vi "Wavelength2Color.vi"(8 "error in (no error)":errorcluster, 11 "Wavelength":u16=380 min=350 max=850 step=1) -> (0 "error out":errorcluster, 3 "Color":u32(colorbox))   [LabVIEW 2023]
doc: "This vi converts a wavelength into a color"
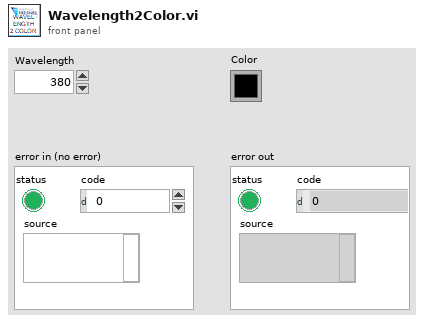
[diagram p1: front panel]
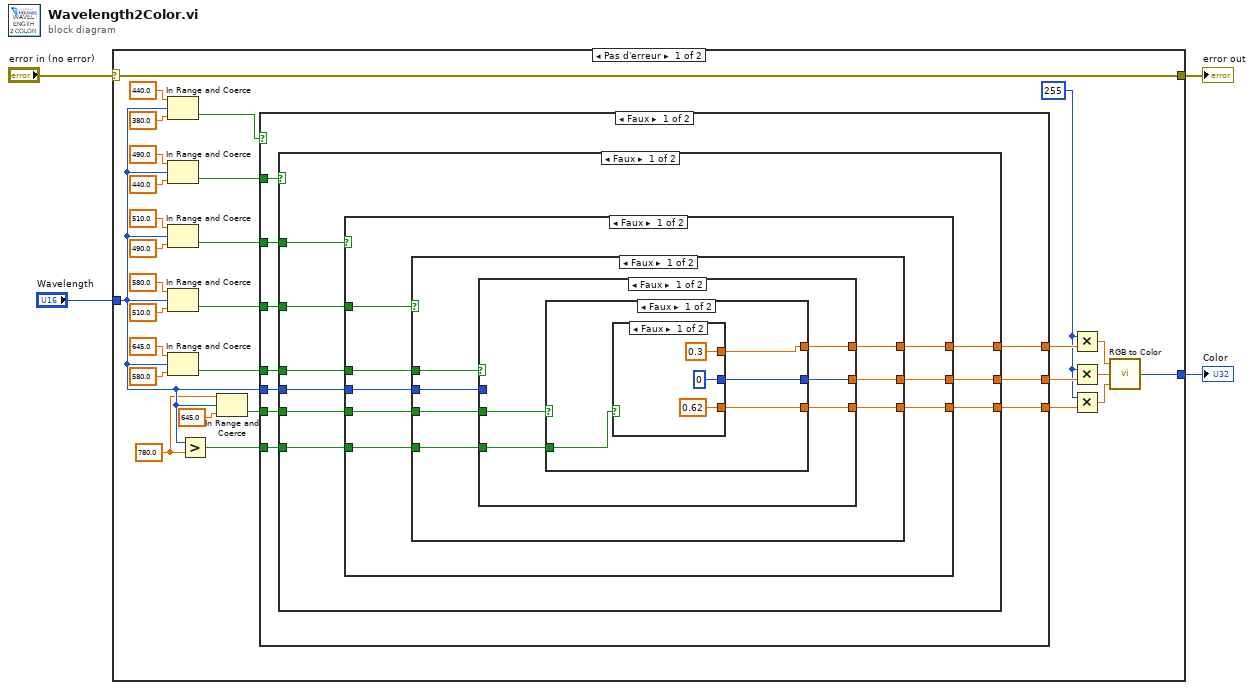
[diagram p0: block diagram]
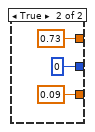
[diagram p2: hidden frame]
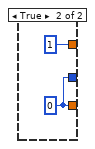
[diagram p3: hidden frame]
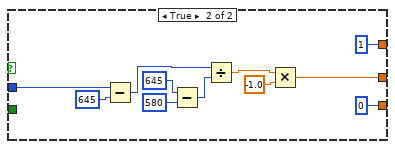
[diagram p4: hidden frame]
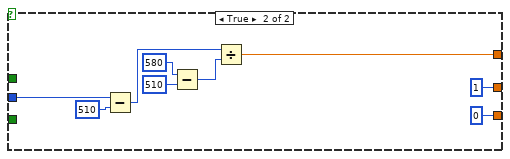
[diagram p5: hidden frame]
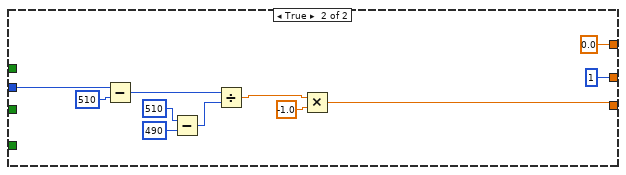
[diagram p6: hidden frame]
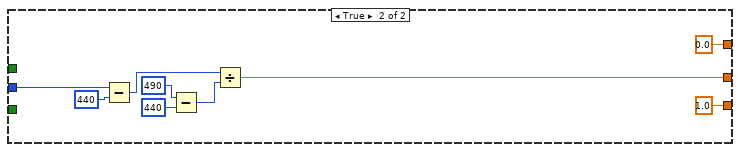
[diagram p7: hidden frame]
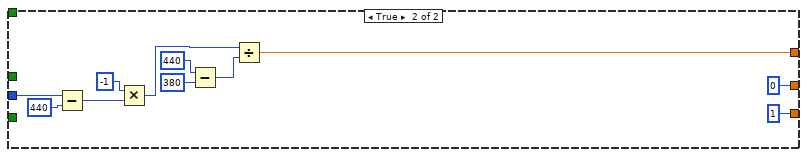
[diagram p8: hidden frame]
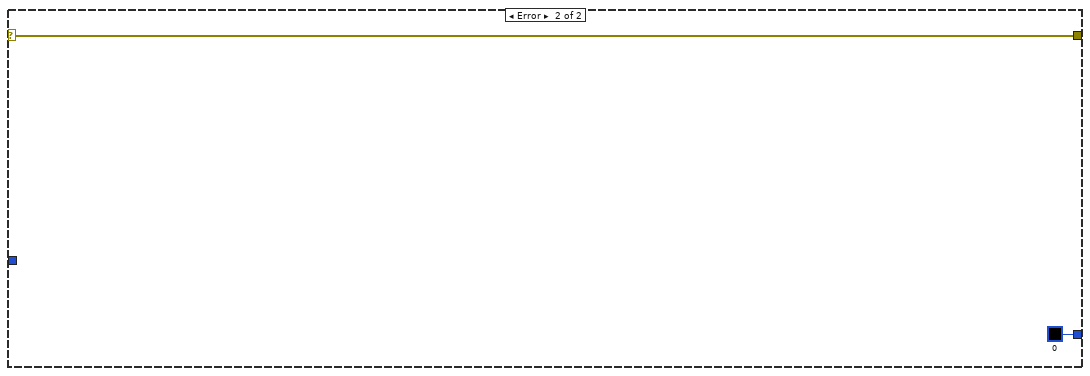
[diagram p9: hidden frame]
diagram:
  n1 = case shown="Pas d'erreur" "error in (no error)" {
    selector: "error in (no error)" -> [w8 w137]
    tunnel: [w8 w137] -> w4
    tunnel: "Wavelength" -> [w7 _]
    tunnel: [w9 u32 0 ("Color")] -> w1
    frame No Error {
      w21 = 255
      w6 = 780.0 ("upper limit")
      n2 = In Range and Coerce(upper limit=440.0, x=w7, lower limit=380.0) -> (In Range?=w22:bool)  [unwired: 1 out]
      n3 = In Range and Coerce(upper limit=490.0, x=w7, lower limit=440.0 ("upper limit")) -> (In Range?=w23:bool)  [unwired: 1 out]
      n4 = In Range and Coerce(upper limit=510.0, x=w7, lower limit=490.0 ("upper limit")) -> (In Range?=w24:bool)  [unwired: 1 out]
      n5 = In Range and Coerce(upper limit=580.0, x=w7, lower limit=510.0 ("upper limit")) -> (In Range?=w25:bool)  [unwired: 1 out]
      n6 = In Range and Coerce(upper limit=645.0, x=w7, lower limit=580.0 ("upper limit")) -> (In Range?=w26:bool)  [unwired: 1 out]
      n7 = Greater?(x=w7, y=w6) -> (0:w5:bool)
      n8 = In Range and Coerce(upper limit=w6, x=w7, lower limit=645.0 ("upper limit")) -> (In Range?=w27:bool)  [unwired: 1 out]
      n9 = case shown="Faux" w22 {
        tunnel: w23 -> [w43 _]
        tunnel: w24 -> [w42 _]
        tunnel: w25 -> [w41 _]
        tunnel: w26 -> [w40 _]
        tunnel: w27 -> [w39 _]
        tunnel: w7 -> [w35 w134]
        tunnel: [w38 w128] -> w28
        tunnel: [w36 0] -> w29
        tunnel: [w37 1] -> w30
        tunnel: w5 -> [w34 _]
        frame False {
          n10 = case shown="Faux" w43 {
            tunnel: w42 -> [w52 _]
            tunnel: w41 -> [w51 _]
            tunnel: w40 -> [w50 _]
            tunnel: w39 -> [w49 _]
            tunnel: [w48 0.0] -> w38
            tunnel: [w46 1.0] -> w37
            tunnel: [w47 w119] -> w36
            tunnel: w35 -> [w45 w118]
            tunnel: w34 -> [w44 _]
            frame False {
              n11 = case shown="Faux" w52 {
                tunnel: w51 -> [w60 _]
                tunnel: w50 -> [w59 _]
                tunnel: w49 -> [w58 _]
                tunnel: [w56 0.0] -> w48
                tunnel: [w55 1] -> w47
                tunnel: [w54 w107] -> w46
                tunnel: w45 -> [w57 w109]
                tunnel: w44 -> [w53 _]
                frame False {
                  n12 = case shown="Faux" w60 {
                    tunnel: w59 -> [w67 _]
                    tunnel: w58 -> [w66 _]
                    tunnel: w57 -> [w65 w99]
                    tunnel: [w63 w98] -> w56
                    tunnel: [w64 1] -> w55
                    tunnel: [w62 0] -> w54
                    tunnel: w53 -> [w61 _]
                    frame False {
                      n13 = case shown="Faux" w67 {
                        tunnel: w66 -> [w72 _]
                        tunnel: w65 -> [_ w89]
                        tunnel: [w70 w87] -> w64
                        tunnel: [w71 1] -> w63
                        tunnel: [w69 0] -> w62
                        tunnel: w61 -> [w68 _]
                        frame False {
                          n14 = case shown="Faux" w72 {
                            tunnel: [w73 1] -> w71
                            tunnel: [w74 w83] -> w70
                            tunnel: [w75 w83] -> w69
                            tunnel: w68 -> [w76 _]
                            frame False {
                              n15 = case shown="Faux" w76 {
                                tunnel: [0.62 0.09] -> w75
                                tunnel: [u8 0 0] -> w74
                                tunnel: [0.3 0.73] -> w73
                                frame False {
                                }
                                frame True {
                                }
                              }
                            }
                            frame True {
                              w83 = 0
                            }
                          }
                        }
                        frame True {
                          n16 = Subtract(x=w89, y=645) -> (x-y=w95:i32)
                          n17 = Subtract(x=645, y=580) -> (x-y=w93:i32)
                          n18 = Divide(x=w95, y=w93) -> (x/y=w88:dbl)
                          n19 = Multiply(x=w88, y=-1.0) -> (x*y=w87:dbl)
                        }
                      }
                    }
                    frame True {
                      n20 = Subtract(x=w99, y=510) -> (x-y=w104:i32)
                      n21 = Subtract(x=580, y=510) -> (x-y=w102:i32)
                      n22 = Divide(x=w104, y=w102) -> (x/y=w98:dbl)
                    }
                  }
                }
                frame True {
                  n23 = Subtract(x=w109, y=510) -> (x-y=w115:i32)
                  n24 = Subtract(x=510, y=490) -> (x-y=w113:i32)
                  n25 = Divide(x=w115, y=w113) -> (x/y=w106:dbl)
                  n26 = Multiply(x=w106, y=-1.0) -> (x*y=w107:dbl)
                }
              }
            }
            frame True {
              n27 = Subtract(x=w118, y=440) -> (x-y=w122:i32)
              n28 = Subtract(x=490, y=440) -> (x-y=w120:i32)
              n29 = Divide(x=w122, y=w120) -> (x/y=w119:dbl)
            }
          }
        }
        frame True {
          n30 = Subtract(x=w134, y=440) -> (x-y=w133:i32)
          n31 = Multiply(x=-1, y=w133) -> (x*y=w132:i32)
          n32 = Subtract(x=440, y=380) -> (x-y=w129:i32)
          n33 = Divide(x=w132, y=w129) -> (x/y=w128:dbl)
        }
      }
      n34 = Multiply(x=w21, y=w28) -> (x*y=w31:dbl)
      n35 = Multiply(x=w21, y=w29) -> (x*y=w32:dbl)
      n36 = Multiply(x=w21, y=w30) -> (x*y=w33:dbl)
      n37 = call <vilib>:"RGB to Color.vi"("B"=w33, "G"=w32, "R"=w31) -> ("Color"=w9:u32)
    }
    frame Error {
    }
  }
  "Color" <- w1
  "error out" <- w4
